vi "wariancja(SubVI).vi"(6 "iteracja N":i32, 7 "wariancja N-1":dbl, 9 "œrednia N-1":dbl, 10 "Gaussian white noise":dbl, 11 "œrednia N":dbl) -> (3 "wariancja":dbl)   [LabVIEW 2025]
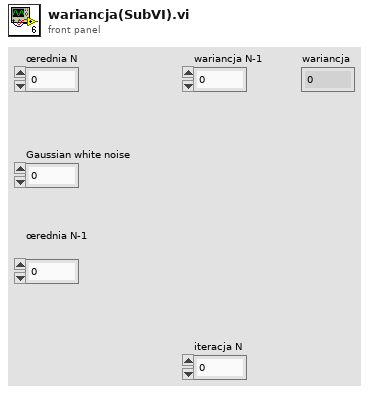
[diagram p1: front panel]
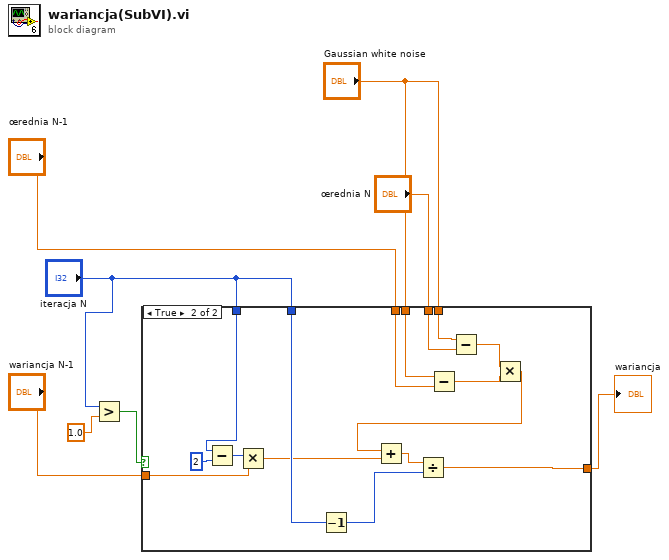
[diagram p0: block diagram]
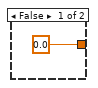
[diagram p2: hidden frame]
diagram:
  n1 = Greater?(x="iteracja N", y=1.0) -> (0:w2:bool)
  n2 = case shown="True" w2 {
    tunnel: "iteracja N" -> [_ w22]
    tunnel: "wariancja N-1" -> [_ w21]
    tunnel: "iteracja N" -> [_ w19]
    tunnel: [0.0 w18] -> w8
    tunnel: "œrednia N" -> [_ w14]
    tunnel: "Gaussian white noise" -> [_ w13]
    tunnel: "œrednia N-1" -> [_ w12]
    tunnel: "Gaussian white noise" -> [_ w11]
    frame False {
    }
    frame True {
      n3 = Subtract(x=w19, y=2) -> (x-y=w23:i32)
      n4 = Multiply(x=w23, y=w21) -> (x*y=w17:dbl)
      n5 = Decrement(x=w22) -> (x-1=w25:i32)
      n6 = Subtract(x=w11, y=w12) -> (x-y=w16:dbl)
      n7 = Subtract(x=w13, y=w14) -> (x-y=w15:dbl)
      n8 = Multiply(x=w15, y=w16) -> (x*y=w10:dbl)
      n9 = Add(x=w10, y=w17) -> (x+y=w24:dbl)
      n10 = Divide(x=w24, y=w25) -> (x/y=w18:dbl)
    }
  }
  "wariancja" <- w8
